vi "2023_day13_Task1.vi"() -> ()   [LabVIEW 2021]
panel:
  out "Task 1":i32
  in  "Switch":bool caption="Ex. Data  vs.  User Data"
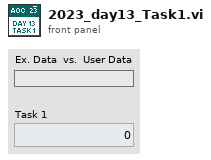
[diagram p1: front panel]
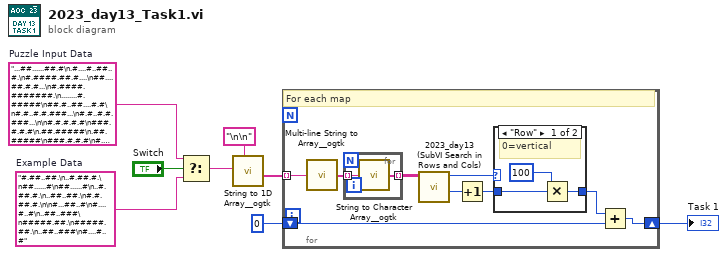
[diagram p0: block diagram]
diagram:
  w6 = "...##......##.#\n.#....#..##..#.\n#.####.##.#....\n##....##.#.#...\n#.####.#######.\n........#.#####\n##.#..##....#.#\n#.#..#.#.###...\n#.#..#.#.###...\n\n#.#.#.#.#\n###.#.#.#\n.##.#####\n.##.#####\n###.#.#.#\n#.#.#.#.#\n.#.##.#.#\n#.#..#..#\n..###.#..\n#..#.#.#.\n##.#...#.\n\n##.....#...\n##.....#...\n#..###....#\n##.#..#.##.\n#..#####..#\n#.#....#.#.\n.##.##....#\n.###..###.#\n...#.......\n....#.#.###\n#......#.##\n...#.##....\n...#.##....\n#......#.##\n....#.#.###\n...#.......\n.###..#####\n\n..####....#\n..####....#\n..#....#.##\n.....#.#..#\n#.#...##...\n###.###.##.\n..#..#...##\n..#..#...##\n###.###.##.\n#.#...##...\n.....#.#..#\n..#.#..#.##\n..####....#\n\n#.#####..\n#..#.#.#.\n.##.#..#.\n.##...##.\n.....#.##\n........#\n........#\n\n..#.###.##..#\n.##.###.##..#\n.#...#.#.#.##\n.#...#.#.#.##\n.##.###.##..#\n..#.###.##..#\n...#.#####.#.\n##.#...######\n..#..#..##.#.\n#..####.###.#\n.##..#....###\n\n####.##....\n....##.##.#\n...##...##.\n##..#..#..#\n##..#....#.\n##..#....#.\n##..#..#..#\n...##...##.\n....##.##.#\n####.##....\n##..#####..\n#..#....#..\n...#.....##\n....#####..\n########...\n#######.#.#\n####.#.#...\n\n..##.......\n#..##.#..#.\n.##....##..\n.#####....#\n#######..##\n.#...##..##\n..####.##.#\n#####..##..\n##.....##..\n##.....##..\n.####..##..\n\n#.#..###.#.##.#\n##.##.###.#..#.\n##...#..#......\n.##...##...##..\n##...###.#.##.#\n.##...#..######\n.#.###.....##..\n...###....#..#.\n#..##..##.#..#.\n#..##..##.#..#.\n...###....#..#.\n.#.###.....##..\n.##......######\n\n#.####.\n#..##..\n##.##.#\n...##..\n#.#..#.\n#####.#\n..#..#.\n..#..#.\n#####.#\n#.#..#.\n...##..\n##.##.#\n#..##..\n#.####.\n..####.\n\n..##.####.#..#.##\n..##..###.#..#.##\n....###..#.##.#..\n......##.######.#\n#.#.#.#..#....#..\n##..###...####...\n#..##..#.#....#.#\n\n##.##..##\n##...##.#\n####.#...\n####.#...\n##...##.#\n##.##..##\n.####.##.\n.##.#...#\n....#....\n#.#..#...\n#.#..#..#\n\n##.##.#..#.\n.#.###....#\n#.#####..##\n#.#####..##\n#....#.....\n##..#######\n.####......\n##.#.######\n##.#.######\n.####......\n##..#######\n\n####.##..\n#..##..##\n.....##..\n#..######\n####.##.#\n####....#\n.##..##..\n####....#\n#..##..##\n.##.#..#.\n#..#.##.#\n.##......\n....####.\n.##..##..\n.....##..\n\n....##..#.#....\n....##..#.#....\n#####.#.#..###.\n.##.#.###.####.\n#.....#..#..###\n.##....#.#....#\n.##.##.#..##..#\n\n.##....##.##..#\n.##.#.#..#...#.\n#..#.#######...\n#..####.##.#..#\n#.##.##.##..#.#\n#..#..#.##..###\n#..#..#.##..###\n\n######...##\n.#####...##\n#.#####..##\n#.#.#.#.#..\n###.#..#...\n..#.....##.\n#....##.##.\n#....##.##.\n..#.....##.\n###.#..#...\n#.#.#.#.#..\n\n...##.....#\n.##...##...\n.##...##...\n.##...##...\n.##...##...\n...##.....#\n.#######.#.\n#...#..##..\n.....##.#.#\n.#.#.#.###.\n.#.#.#.###.\n.....##.#.#\n#...#..##..\n.##.####.#.\n...##.....#\n\n.##.##.\n.##...#\n....###\n#..#...\n#..#.##\n.....##\n#..##..\n.#...##\n#..#.##\n.##.##.\n.##..##\n.##..##\n.##.##.\n\n.##.###........\n##.#.####.##.##\n.####...#.##.#.\n#.##......##...\n...###...####..\n.#.......#..#..\n.#.#..#...##...\n\n##..##.##..#.\n.####......#.\n......#.#####\n.####...#.#..\n.#..#.#.##..#\n#.##.##.#.##.\n.#..#..#..##.\n######.#.#...\n#....###...#.\n#....###...#.\n######.#.#...\n.#..#..##.##.\n#.##.##.#.##.\n\n###..####\n##.##.###\n.######..\n...##....\n...##....\n.#....#..\n##....###\n.##..##..\n##....###\n###..##..\n#.#..#.##\n\n..##..##.\n.#.#.##.#\n.###.##.#\n..##..##.\n..#.#.#..\n#.##....#\n..####..#\n###..#.##\n#...##...\n#...##...\n###..#.##\n\n####.##.#######\n#...####...####\n##.######.#####\n##.######.##...\n..#......#...##\n###.####.######\n####...######..\n#..#.##.#..####\n#.##.##.##.##..\n.##.####.##.#..\n#....##....####\n..#.#..#.#...##\n##..####..##...\n\n...#.#.....##..\n####.#.#.......\n#.#....##..##..\n..#..#.....##..\n.##.#...#..##..\n#.#..##........\n...##..########\n#######.#..##..\n##.####..######\n###...###.####.\n#........######\n.#.##..........\n..##..#.###..##\n.#.#.#..#..##..\n.....###.##..##\n#...#.##.......\n##..##..#......\n\n#..###.....##\n...#...#...##\n##.#.##.....#\n..###..###.##\n.###..##...##\n###.#######..\n#.###...##..#\n#..##...##..#\n###.#######..\n.###..##...##\n..###..###.##\n##.#.##.....#\n...#...#...##\n#..###.....##\n.#.##.##.##..\n.#.##.##.##..\n#..###.....##\n\n##...##.#..#.\n##...##......\n###..##..##..\n###.#........\n....#########\n....#########\n###.#........\n###..##..##..\n#....##......\n##...##.#..#.\n##...#..####.\n..#.##.......\n#.##.########\n#.#.##.##..##\n##...#..####.\n\n.#.##....##.##.\n#####.####..#.#\n.#....##..###.#\n.#...#######..#\n..##.##.#....#.\n...#.#..##.#..#\n...#.#..##.#..#\n..##.##.#....#.\n.#.#.#######..#\n.#....##..###.#\n#####.####..#.#\n.#.##....##.##.\n...#.#.##.##...\n..#.#.#.#.#.###\n##...#.#.....##\n##...#.#.....##\n..#.#.#.#.#.###\n\n..#....#....##...\n##..##..#########\n.#......#.##..##.\n###.##.###..##..#\n##############.##\n.########.#.##.#.\n#..####..#.####.#\n...#..#..........\n#.######.##.##.##\n.##....##...##...\n#..####..#..##..#\n\n#.##.#####.##..#.\n#....#.###...##..\n#....#.##..###..#\n#....#.##..###...\n#....#.###...##..\n#.##.#####.##..#.\n#######..#.####..\n.........#..#....\n########.#...#.##\n#....#.###..#.##.\n##..###..#.#..###\n#....#...###.....\n.####..#.#.#.....\n######..##....###\n######.###...#.#.\n\n.#..#.########.#.\n.####..######..#.\n#....##......##..\n.####.#..##..#.##\n##..#####..#####.\n######..#..#..###\n#########..######\n.####...#..#...##\n######...##...###\n#....#..#..#..#..\n......###..###...\n.#..#.#.####.#.#.\n#.##.##.####.##.#\n.####.#......#.##\n##..##.##..##.##.\n\n.##.#.#..\n#.###....\n###......\n...#.####\n##...##..\n##..#..##\n###.#....\n###.#....\n##..#..##\n##...##..\n...#.####\n###......\n#.###.#..\n.##.#.#..\n.######..\n\n####....##.##.#\n..##.##..##.#.#\n..##.##..##.#.#\n####..#.##.##.#\n..##.#........#\n#.....##....###\n#.#..##...#....\n.###..#..##.##.\n#..#.#.#..##.#.\n##.####.#####..\n..##..#.##...##\n#.##...##.#.#.#\n#..#.##..###..#\n#.##.######...#\n#.##.######...#\n\n##.##.##.\n..####...\n..####..#\n########.\n...##...#\n..####..#\n..####..#\n.#....#..\n..####...\n##.##.###\n###..####\n..####..#\n........#\n##....###\n##....###\n..#..#..#\n..####...\n\n..########.\n..########.\n#.#..###..#\n.#...#.....\n..#...#....\n.#.##..#..#\n.#.....#..#\n.....###...\n#..####.##.\n#..####.##.\n.....###...\n.#.....#.##\n.#.##..#..#\n..#...#....\n.#...#.....\n#.#..###..#\n..########.\n\n....##....#\n..###.#..#.\n.###.######\n.###.######\n..###.#..#.\n....##....#\n##..##.##.#\n.###..#..#.\n##...#.##.#\n.##.#######\n..#.##.....\n.###.......\n#######..##\n##.#.##..##\n#..##.####.\n\n..###..#......#\n##..#.##.#..#.#\n...#.##..#..#..\n..###.####..###\n#####.#..####..\n...#..###.##.##\n..#.#.###..#.##\n##..#..########\n..##.#.########\n.....###..##..#\n..#.##.#......#\n####.#.##.##.##\n########.#..#.#\n..####.##.##.##\n..#.##..#....#.\n\n#.####.#.####.#\n..#..#...##.##.\n.##..##.#......\n.##..##.#......\n..#..#..###.##.\n#.####.#.####.#\n########....##.\n.#.##.#..##..##\n.#.##.#.#.##..#\n#..##..#.##...#\n............#.#\n##....###.....#\n#.#..#.#.###.##\n\n..######......#\n.########.##.##\n..#.##.#......#\n..#.##.#......#\n#.#....#.#..#.#\n##.####.######.\n###...####..###\n\n...#.#.##..#...##\n..#.#.#.########.\n....#....##.#....\n##.......#.....##\n##...##...#.#..##\n.#.#####.#....#..\n.....#####.##.#..\n##.#....#..###...\n.#.#.##...####.##\n.....######..##..\n#.##..#....#.##..\n##.....#...###...\n#.##..#..#.##..##\n#.##..#..#.##..##\n##.....#...###...\n\n#.###..##\n.#.#....#\n##.#..#..\n.##.#..##\n####.....\n.###.....\n.#...#.##\n..#...#..\n..#.#####\n.#.#.....\n.#.#.....\n..#.#####\n..#...#..\n.#...#.##\n.###.....\n\n..##...#.##.#...#\n#.#.##...##...##.\n##.....#....#....\n..#.##........##.\n###.##.#.##.#.##.\n##..##..#..#..##.\n########....#####\n.#.....##..##....\n###.##.##..##.##.\n\n##..#.##....#\n.##..###....#\n#.#.#....##..\n#.##.#..####.\n#.#.#.##....#\n#..####......\n#..####......\n#.#.#.##....#\n#.##.#..####.\n#.#.##...##..\n.##..###....#\n\n...###....#\n...###....#\n..##..#.#..\n..#.....#..\n.........#.\n###..#.##.#\n##.#..#.###\n.#.........\n###.##..#..\n..#.##.####\n##...###.##\n##..#...#..\n##.#.##.##.\n....#..##..\n...#.#####.\n\n.####..#.##..##..\n.###....###..##..\n#.#.#..#.#.#....#\n#####..#####.##.#\n##.##..##.##.##.#\n###......####..##\n##.#.##.#.##.##.#\n\n.#....##.#....#\n.#.##.#.#####..\n###..#.###.###.\n#...#.#.#..###.\n.##.##..#....#.\n###.#.#.#.##..#\n###..#..#..#.#.\n###..#..#..#.#.\n###.#.#.#.##..#\n.##.##..#....#.\n#...#.#.#..###.\n###..#.###.###.\n.#.##.#.#####..\n.#....##.#...##\n.#....##.#...##\n\n###...#..#.#.#.\n.....#.####.#.#\n####..#.#..#.##\n#.#..##.###.###\n##.#####.###.##\n##.#####.###.##\n#.#..##.###.###\n###...#.#..#.##\n.....#.####.#.#\n###...#..#.#.#.\n...#.###.#...##\n.##.#......####\n.##.#......####\n...#.###.#...##\n###...#..#.#.#.\n\n..######..#\n###.##.####\n##.####.##.\n.##....##.#\n##.####.###\n...#..#...#\n###....###.\n..#.##.#..#\n..##..##...\n..##..##...\n##..##..##.\n...#..#....\n###.##.####\n##.####.##.\n....##....#\n\n##.#....#.#\n..#......#.\n##...##...#\n##........#\n##.######.#\n..##.##.###\n...######..\n....#..#...\n..#.####.#.\n..#.#..#.#.\n###.####.##\n...#.##.#..\n##..#..#..#\n..#..##..#.\n##.######.#\n\n###.##..#\n.#####..#\n....#....\n###...##.\n##.##.##.\n####.....\n..###....\n\n##.##.##.##\n##.########\n...#......#\n####..##..#\n##..#....#.\n###.######.\n##.##....##\n##.#..##..#\n##.#.####.#\n##..#....#.\n######..###\n##.........\n###..####..\n..#.#.##.#.\n###..#..#..\n...###.####\n#####.##.##\n\n.#..######..#..#.\n#..###..###..##..\n#...######...##..\n..###....#.#....#\n#....####....##..\n.##..####..##..##\n.#.##....##.#..#.\n###.#.##.#.######\n##..##..##..####.\n#.#..#..#..#.##.#\n...#..##..#......\n\n##.#..#\n###...#\n.###.##\n.###.##\n###...#\n##.#..#\n..#..##\n##..#..\n.#.....\n.#.....\n##..#..\n#.#..##\n##.#..#\n\n####.#.\n..#...#\n##...#.\n..#..##\n###.##.\n....#..\n##.####\n##....#\n..#####\n..#####\n##....#\n##.####\n....#..\n###.##.\n..#..##\n##...#.\n..#.#.#\n\n..##.###.##.###\n#..#.##.####.##\n##.##..######..\n###..##.####.##\n.####..........\n..##..########.\n.##..##......##\n.##..##......##\n..##..########.\n.####..........\n###..##.####.##\n##.##..######..\n#..#.##.####.##\n..######.##.###\n#....#.#.##.#.#\n\n#####..\n##.#.##\n..#####\n.##..##\n..#..##\n...#.##\n##.##..\n.####..\n##.....\n.#..#..\n.#..#..\n##.....\n..###..\n##.##..\n...#.##\n\n..####.##.#\n.#.##.#..#.\n.#....#....\n.######...#\n##.##.##...\n.######...#\n.#....#.##.\n###..###..#\n##....#####\n..#..#...#.\n..#..#...#.\n\n###..#.\n...###.\n.##.###\n.#####.\n##..###\n.###.##\n.#..#..\n..###..\n..###..\n.#..#..\n####.##\n##..###\n.#####.\n.##.###\n...###.\n###..#.\n###..#.\n\n..#######\n...######\n...##....\n##.#..###\n..#.#.###\n.##....##\n######...\n#..######\n.#.####..\n.#..##...\n..###....\n.#####.##\n##.###...\n\n...##....##\n...##....##\n#.####.#...\n.#.##.#.##.\n.#....#.###\n.######..#.\n.........##\n..####....#\n.#....#...#\n...##...#.#\n##.##.####.\n#..##.##...\n#.#..#.##..\n\n######...#....#\n..##...........\n..##..#.##.##.#\n##..####.#.##.#\n#.##.##.#.####.\n.####..##.####.\n########.######\n#.##.##.###..##\n.#..#..#.#.##.#\n.####.#.#......\n#.##.#...####.#\n\n#...#.###\n.###..##.\n..##.#.##\n.##.#.#..\n..#.##.#.\n.#..#..#.\n.#.#.#.##\n.#.###.##\n.#..#..#.\n.#..#..#.\n.#.###.##\n.#.#.#.##\n.#..#..#.\n\n....#.##..###\n#######.#.#..\n##.#..##.....\n####.#.#.#.##\n#####......##\n...###.###.#.\n......####.##\n\n.#..###..###..#..\n.#.#..#..#..#.#..\n.#..##.##.##..#..\n.......##........\n##.##.#..#.##.###\n###..######..####\n##.##.#.##.##.###\n#.#..######..#.##\n..#...####...#...\n\n#....#....#\n.####....#.\n#....##.#..\n#....####..\n.####....#.\n#....#....#\n.####....##\n\n########.\n##.##.###\n...##...#\n..####..#\n#.#..#.#.\n##....###\n##....###\n###..###.\n###..###.\n...##...#\n...##...#\n..####...\n........#\n\n#.###..##\n##...##..\n#.#......\n#....##..\n#....##..\n..#.####.\n..#......\n\n..#..###...#.\n..#..###...#.\n...##...##.##\n##....##...#.\n##.##.##.#..#\n...######...#\n..#..#...#.##\n##...##..#...\n#..#.##..#..#\n....#.#.#.##.\n###..#.#.##.#\n\n#..#...\n...##.#\n.#.....\n..#.#.#\n..#.#.#\n.#.....\n...####\n#..#...\n#.#.#.#\n#.#.#.#\n#..#...\n...####\n.#.....\n\n..##.####.##...##\n..##.####.##...##\n..#..#..#..#..##.\n.##.##..##.##.#..\n#...##..##...#.#.\n#.##......##.#.#.\n.##..#..#..##.#..\n#...##..#....####\n######..#######.#\n.###.####.###..#.\n.##..####..##.#..\n\n##.#.######..#.##\n.##..#..#.###.#..\n#####..#####...##\n#####..#####...##\n.##..#..#.###.#..\n##.#.######..#.##\n.##.###....###.##\n.##..####..#....#\n.##.####.#.#.####\n..#..#.#...####..\n.###...######.###\n\n...#.#.###.\n...#.#.###.\n###...##.##\n......##..#\n#.#..#..#..\n.#.#..#...#\n##.##..##..\n#..#.#..##.\n#..###..#..\n#.####..#..\n#..#.#..##.\n\n#.#....#...\n.#.###.###.\n..##.##...#\n.#..###..##\n..#...#..##\n..#...#..##\n.#..###..##\n..##.##...#\n.#.##..###.\n#.#....#...\n...#####...\n...#####...\n#.#....#...\n.#.##..###.\n..##.##...#\n\n#.#####..#.#.#.#.\n##..#..#.##.##..#\n..##......#...#..\n####...###.#.#.#.\n...#.#.#....#####\n....#....##.##.#.\n....#....##.##.#.\n#..#.#.#....#####\n####...###.#.#.#.\n..##......#...#..\n##..#..#.##.##..#\n#.#####..#.#.#.#.\n#.#####..#.#.#.#.\n\n#.#..##..##.#\n##..#...###..\n#.##.#....#..\n#.##.#....#..\n##..#...###..\n#.#..##..#..#\n##.##.#..#..#\n...#######.#.\n.###.##....##\n.#.#....#...#\n.##.##..##...\n###.#.#.#.###\n###.#...###..\n.#.###.....#.\n#.#.####..##.\n#.#.####..##.\n.#.###.....#.\n\n.##..#.####..\n.#.#.#.######\n#.###..###...\n#..##.#.#####\n###..#.#.#.#.\n#.##.#.##.###\n...#.###.####\n##.#.##....##\n##.#.##.#..##\n.#.#..####.##\n##.###..#..#.\n##.###..#..#.\n.#.#..####.##\n##.#.##.#..##\n##.#.##....##\n\n#...##..#\n#####....\n#####....\n#...##..#\n.#....###\n.#.#..###\n#...##..#\n\n#......##\n#......#.\n.##..##..\n.##..##..\n#......##\n###..####\n#......##\n#.#..#.##\n##.##.###\n..#..#..#\n........#\n..####...\n.#.##.#..\n........#\n........#\n.#.##.#..\n.######..\n\n#........#..#..#.\n##..##..##..##..#\n#..####..####..##\n#.#....#.#..#.#..\n.#......#.##.#...\n.##....##.##.##..\n##.#..#.######.#.\n###.##.########.#\n..#....#..##..#..\n\n..........###..##\n####..#######.#..\n##.#..#.###....##\n#........#.###...\n####..####.#...##\n.##....##.##.#...\n##.####.##..###..\n###.##.###...##..\n##.####.##.##.###\n.#..##..#.###..##\n##..##..###.##...\n.########.#.##.##\n.#.####.#...###..\n.###..###.#######\n#.#.##.#.##...#.#\n..#.##.#..##.#.##\n#........###.##..\n\n..#.###\n.#.....\n..#.##.\n..#.##.\n.#.....\n..#.###\n#.####.\n.##...#\n.#.###.\n.#.###.\n.#....#\n\n#..###.\n####..#\n####..#\n#..###.\n.##.##.\n###.###\n...####\n...####\n###.###\n.#..##.\n#..###.\n\n#....#...#...\n#....#.####.#\n#....#.####.#\n#....#...#...\n......######.\n.####.#..##.#\n#######..#.##\n.##.#..##.#.#\n#....######.#\n\n..#....#.##..##\n.#....####.##..\n.#.##...#######\n#.##..###......\n#.#.....#######\n##.#.....######\n###...##...##..\n..##..##.#....#\n###.##...#....#\n..###.##.......\n#.##...##......\n.##...###.#..#.\n.##...###.#..#.\n#.##...##......\n..###.##.......\n###.##...#....#\n..##..##.#....#\n\n....#...#.#.#..\n##...#.#.#.....\n.####.##.......\n.......#.#.##.#\n#..#..#.#..#.#.\n#..##.#.#..#.#.\n.......#.#.##.#\n.####.##.......\n##...#.#.#.....\n....#...#.#.#..\n....#...#.#.#..\n\n#..####..#..#\n#..#..#..####\n#..#.....#..#\n##..##..#####\n#..####..#..#\n##..##..##..#\n.###..###....\n\n..#....##\n...##..#.\n...######\n##.#.#..#\n######.#.\n......#.#\n#####.##.\n...##....\n##.##.##.\n...##....\n##..#####\n##..#####\n...##..#.\n##.##.##.\n...##....\n#####.##.\n......#.#\n\n####.###.\n####..#..\n####..#..\n####.###.\n#..#.####\n......##.\n#..#.##..\n....#.##.\n#..#..###\n##.##..##\n.##......\n\n###.#.#.#\n###.#.#.#\n...#.#.##\n#.##..#..\n#.###.##.\n#.####.#.\n##.######\n#.##..#..\n#.##..#..\n##.######\n#.####.#.\n#.######.\n#.##..#..\n...#.#.##\n###.#.#.#\n\n...#.#.##.#\n...#.#.##.#\n#.#.#.#...#\n#.###...##.\n#..##.##.##\n##..####.#.\n##..####.#.\n#..##.##.##\n#.####..##.\n\n#.#.#.##.###.\n..##.#..##...\n..##.#..##...\n..#.#.##.###.\n.#.#.##....#.\n..#.#.###.#.#\n..#.#.###.#.#\n\n...#......#..\n##...#..#...#\n###..#..#..##\n...#.####.#..\n..##.#..#.##.\n....######...\n....##...#...\n\n....#.##.########\n.####.##.##......\n..##..###.#.#.#.#\n########....#.##.\n..##......#.#.##.\n.#..#...#..###.##\n.#..#...#..###.##\n\n##...#..###\n..##....###\n....#..#...\n#####..#...\n##.#..####.\n##.#..####.\n#####..#..#\n\n#.###..##.###..\n#....#..##.####\n#.#####.##.#...\n..#####.....#..\n###.####..#####\n##.#.....#.#...\n#.#....##..####\n##..#...#..##..\n.#...#.#..##.##\n##..#.##.##.#..\n#.#.#####.#....\n##..##.#..#....\n.#..##.....##..\n#..#...#...#...\n#.##...#...#...\n..##.#....#.###\n..##.#...##.###\n\n##..###..#.####\n.###.#.##..####\n###...#..#.....\n.........##.##.\n..#....##.#.##.\n###...#...#....\n..#..#....##..#\n#.....#.##.....\n#...#...#......\n.#..##..###....\n.#.###..###....\n\n.##.#..#.....\n########.....\n###..#...####\n####.#.##.##.\n......#.#.##.\n#..#.##.#.##.\n####.##.#####\n.....#..#####\n.##..##.#.##.\n.##...##.####\n.....##.#####\n.##....###..#\n.##.#.#...##.\n.##.#.#......\n#..#..##..##.\n....##.......\n####.#..#....\n\n.###.##.#\n.###.##.#\n##.#.....\n####.##.#\n##...####\n....###..\n.#....#..\n#..#.####\n#..#.####\n.#...##..\n....###..\n##...####\n####.##.#\n##.#.....\n.###.##.#\n\n...#.######\n...#.######\n#.#.#.#....\n###...##...\n##.########\n...#.#.....\n...##.#.##.\n.#...###..#\n..####.####\n.#.#.#.....\n#......####\n\n######...#...\n#.##.##.#####\n######...#...\n.#..#..#####.\n......###..#.\n..##....#.#..\n..##..#.##.##\n..##..#.##.##\n..##....#.#..\n......###..#.\n.#..#..#####.\n######...#...\n#.##.#..#####\n######...#...\n#.##.#.#..###"  # Puzzle Input Data
  w7 = "#.##..##.\n..#.##.#.\n##......#\n##......#\n..#.##.#.\n..##..##.\n#.#.##.#.\n\n#...##..#\n#....#..#\n..##..###\n#####.##.\n#####.##.\n..##..###\n#....#..#"  # Example Data
  n1 = Select(t=w6, s="Switch", f=w7) -> (s? t:f=w5:string)
  n2 = call <userlib>:"String to 1D Array__ogtk.vi"("delimiter (Tab)"="\n\n", "string"=w5) -> ("Array of Strings"=w3:string[])  [unwired: 9 in]
  n3 = for {
    tunnel: w3 -> [w17] mode=indexing
    shift-right: [w12] -> w1
    shift-left: 0 -> [w13]
    # "For each map"
    n4 = call <userlib>:"Multi-line String to Array__ogtk.vi"("string"=w17) -> ("lines"=w16:string[])
    n5 = for {
      tunnel: w16 -> [w19] mode=indexing
      tunnel: [w18] -> w15 mode=indexing
      n6 = call <userlib>:"String to Character Array__ogtk.vi"("Input String"=w19) -> ("Character Array"=w18:string[])
    }
    n7 = call "2023_day13 (SubVI Search in Rows and Cols).vi"("Character Array"=w15) -> ("Match Index"=w9:i32, "Row or Col"=w10:enum32{"Row", "Col"})  [unwired: 8 in, 1 out]
    n8 = Increment(x=w9) -> (x+1=w11:i32)
    n9 = case shown="\"Row\"" w10 {
      tunnel: w11 -> [w22 w23]
      tunnel: [w20 w23] -> w14
      frame "Row" {
        # "0=vertical"
        n10 = Multiply(x=100 ("y"), y=w22) -> (x*y=w20:i32)
      }
      frame "Col", Default {
        # "1=horizontal"
      }
    }
    n11 = Add(x=w14, y=w13) -> (x+y=w12:i32)
  }
  "Task 1" <- w1
